vi "Read LVProject File Path.vi"(8 "error in (no error)":errorcluster, 11 "LangData in":refnum<class "Project Data.lvclass">) -> (0 "error out":errorcluster, 2 "LVProject File Path":path, 3 "LangData out":refnum<class "Project Data.lvclass">)   [LabVIEW 2013, in "SET Project Data.lvlib" / "Project Data.lvclass"]
uses:
  Project Data.lvclass
  Project Data.lvclass/Project Data.ctl
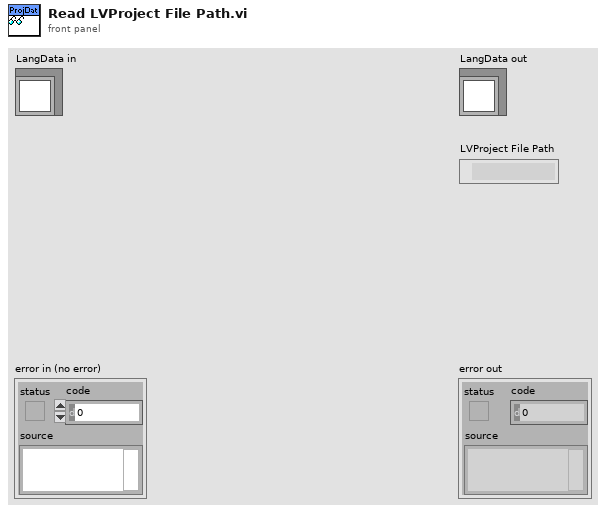
[diagram p1: front panel]
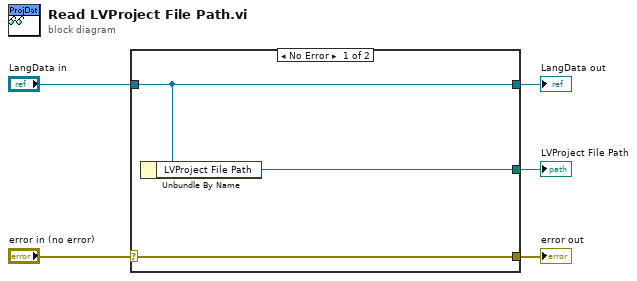
[diagram p0: block diagram]
diagram:
  n1 = case shown="No Error" "error in (no error)" {
    selector: "error in (no error)" -> [w8 w9]
    tunnel: [w8 w9] -> w4
    tunnel: [w7 w10] -> w2
    tunnel: "LangData in" -> [w7 w10]
    tunnel: [w6 _] -> w1
    frame No Error {
      n2 = Unbundle By Name(w7) -> ("LVProject File Path"=w6:path)
    }
    frame Error {
    }
  }
  "error out" <- w4
  "LangData out" <- w2
  "LVProject File Path" <- w1
